vi "Read (Multiple Waveforms).vi"(8 "error in (no error)":errorcluster, 9 "Maximum Time (10000 ms)":u32=10000, 10 "Channels":u16[](array[ring])=[0] items=["Channel 1", "Channel 2", "Channel 3", "Channel 4", "Math 1", "Math 2", "Math 3", "Math 4", "Reference 1", "Reference 2", "Reference 3", "Reference 4"], 11 "VISA resource name":refnum<visa-resource-name>) -> (0 "error out":errorcluster, 2 "Waveform Data":waveform(dbl)[](graph), 3 "VISA resource name out":refnum<visa-resource-name>)   [LabVIEW 2011, in "Tektronix 7000 Series.lvlib"]
doc: "Initiates an acquisition on all channels that you enabled with the Configure Channel VI. This VI waits for the acquisition to complete and returns the waveform for the <B>Channel</B> you specify. If the oscilloscope does not complete the acquisition within the <B>Maximum Time</B> period, this VI returns a timeout error. A timeout error often occurs because the acquisition is not triggered. For example, if the trigger level is out of range of the waveform, the acquisition is not triggered.\n\nRun the Fetch Waveform VI to obtain the waveforms for each of the remaining enabled <B>Channels</B> without initiating another acquisition.\n\n<B>Note:</B> If the instrument does not support autocompensation for probe attenuation, you might need to adjust the scaling of the <B>Waveform Data</B> accordingly. You can adjust the scaling using the Configure Channel VI or manually multiplying the <B>Waveform Data</B> by the probe attenuation."
uses:
  Tektronix 7000 Series.lvlib
  Low Level/Fetch (Waveform).vi
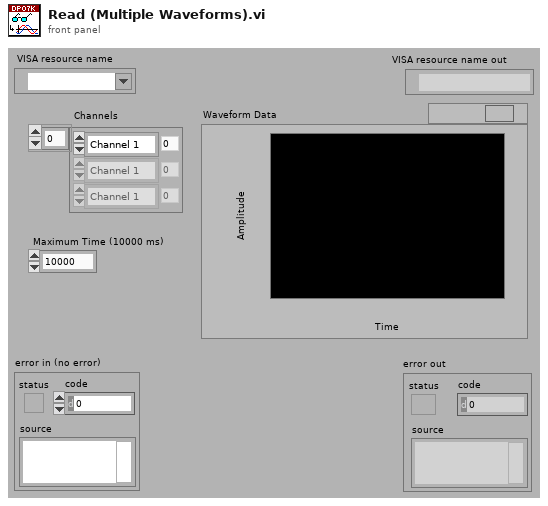
[diagram p1: front panel]
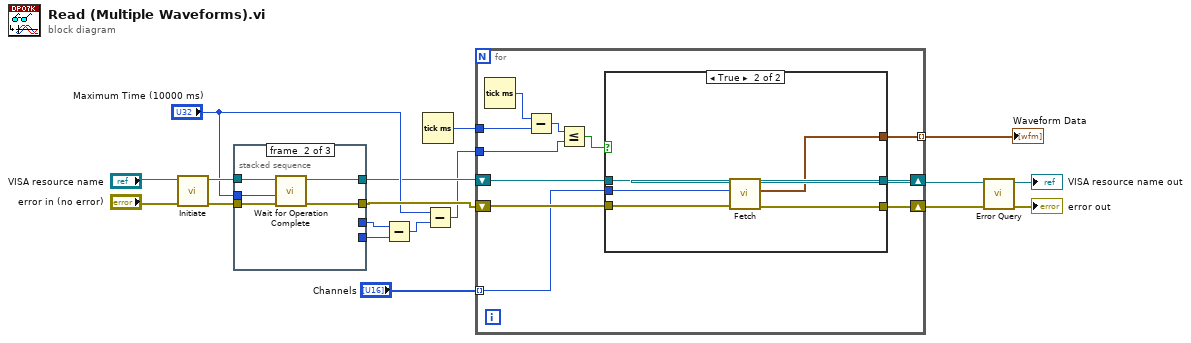
[diagram p0: block diagram]
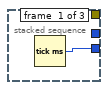
[diagram p2: hidden frame]
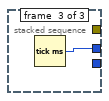
[diagram p3: hidden frame]
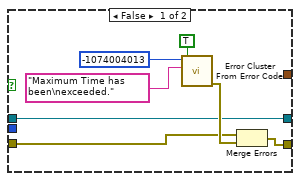
[diagram p4: hidden frame]
diagram:
  n1 = call "Initiate.vi"("error in (no error)"="error in (no error)", "VISA resource name"="VISA resource name") -> ("error out"=w7:errorcluster, "VISA resource name out"=w8:refnum<visa-resource-name>)  [unwired: 8 in]
  n2 = stacked-sequence {
    tunnel: w8 -> [_ w24 _]
    tunnel: w7 -> [_ w23 _]
    tunnel: [_ _ w25] -> w9
    tunnel: [w19 _ _] -> w10
    tunnel: "Maximum Time (10000 ms)" -> [_ w22 _]
    tunnel: [_ w21 _] -> w4
    tunnel: [_ w20 _] -> w6
    frame #0 {
      n3 = Tick Count (ms)() -> (millisecond timer value=w19:u32)
    }
    frame #1 {
      n4 = call "Wait for Operation Complete.vi"("error in (no error)"=w23, "Maximum Time (2000ms)"=w22, "VISA resource name"=w24) -> ("error out"=w20:errorcluster, "VISA resource name out"=w21:refnum<visa-resource-name>)  [unwired: 7 in]
    }
    frame #2 {
      n5 = Tick Count (ms)() -> (millisecond timer value=w25:u32)
    }
  }
  n6 = Subtract(x=w9, y=w10) -> (x-y=w11:u32)
  n7 = Tick Count (ms)() -> (millisecond timer value=w1:u32)
  n8 = Subtract(x="Maximum Time (10000 ms)", y=w11) -> (x-y=w3:u32)
  n9 = for {
    shift-right: [w35] -> w15
    shift-left: w6 -> [w33]
    shift-right: [w36] -> w16
    shift-left: w4 -> [w34]
    tunnel: [w32] -> w12 mode=indexing
    tunnel: w3 -> [w27]
    tunnel: "Channels" -> [w31] mode=indexing
    tunnel: w1 -> [w29]
    n10 = Tick Count (ms)() -> (millisecond timer value=w30:u32)
    n11 = Subtract(x=w30, y=w29) -> (x-y=w28:u32)
    n12 = Less Or Equal?(x=w28, y=w27) -> (x <= y?=w26:bool)
    n13 = case shown="True" w26 {
      tunnel: [w38 w49] -> w36
      tunnel: [w37 w48] -> w35
      tunnel: w34 -> [w38 w47]
      tunnel: w33 -> [w39 w46]
      tunnel: [_ w45] -> w32
      tunnel: w31 -> [_ w44]
      frame False {
        n14 = call <vilib>:"Error Cluster From Error Code.vi"("show call chain? (False)"=TRUE, "error message (\"\")"="Maximum Time has been\nexceeded." ("error message (\"\")"), "error code (0)"=-1074004013) -> ("error out"=w40:errorcluster)  [unwired: 6 in]
        n15 = Merge Errors(w39, w40) -> (w37:errorcluster)
      }
      frame True {
        n16 = call-poly "Fetch.vi"("error in (no error)"=w46, "Channel (0:Channel1)"=w44, "VISA resource name"=w47) -> ("error out"=w48:errorcluster, "Waveform Data"=w45:waveform(dbl), "VISA resource name out"=w49:refnum<visa-resource-name>)  [unwired: 6 in]
      }
    }
  }
  "Waveform Data" <- w12
  n17 = call "Error Query.vi"("error in (no error)"=w15, "VISA resource name"=w16) -> ("error out"=→"error out":errorcluster, "VISA resource name out"=→"VISA resource name out":refnum<visa-resource-name>)  [unwired: 6 in, 2 out]
